vi "getAllChannels.vi"(8 "error in (no error)":errorcluster, 11 "Inst.Krohn-Hite-7008 in":refnum<class "Inst.Krohn-Hite-7008.lvclass">) -> (0 "error out":errorcluster, 2 "allChannelProperties":T1 {"channel" min=1 max=8 step=1}, 3 "Inst.Krohn-Hite-7008 out":refnum<class "Inst.Krohn-Hite-7008.lvclass">)   [LabVIEW 2019, in "Inst.Krohn-Hite-7008.lvclass"]
uses:
  Inst.Krohn-Hite-7008.lvclass
  C:/Program Files (x86)/National Instruments/LabVIEW 2019/user.lib/LevyLab/Instrument Framework/SMOs/Instrument/Instrument.lvclass
  KH7008/typedefs/allChannelProperties--Array.ctl
  KH7008/typedefs/channelProperties--Cluster.ctl
  KH7008/typedefs/channel--numeric.ctl
  KH7008/typedefs/gain--enum.ctl
  KH7008/typedefs/Input--Enum.ctl
  KH7008/typedefs/shunt--enum.ctl
  KH7008/typedefs/couple--Enum.ctl
  KH7008/typedefs/Filter--Enum.ctl
  Typedefs/Inst.Krohn-Hite-7008.PublicCommands--Enum.ctl
  Typedefs/getAllChannelsResponse--Cluster.ctl
  <userlib>/LevyLab/Instrument Framework/SMOs/Instrument/Instrument.lvclass/Instrument.ctl
  38ca2375-f501-4891-9a0c-4469223ebde2.vi
  38ca2375-f501-4891-9a0c-4469223ebde2.vi/5aa567ac-1695-459b-a1d0-b3af6574eea6.vi
  <userlib>/LevyLab/Instrument Framework/SMOs/Instrument/API/Send and Receive.vi
  38ca2375-f501-4891-9a0c-4469223ebde2.vi/e3c320c6-cd25-45d0-953c-8e0f206248d2.vi
  <userlib>/LevyLab/Instrument Framework/SMOs/Instrument/Private/Get Client Type.vi
  38ca2375-f501-4891-9a0c-4469223ebde2.vi/5aa567ac-1695-459b-a1d0-b3af6574eea6.vi/1d0ba0ad-da3a-4e7e-a3ed-5df425220c22.vi
  38ca2375-f501-4891-9a0c-4469223ebde2.vi/5aa567ac-1695-459b-a1d0-b3af6574eea6.vi/db69f284-e81f-4a99-80b8-8d5d4eb5535a.vi
  38ca2375-f501-4891-9a0c-4469223ebde2.vi/e3c320c6-cd25-45d0-953c-8e0f206248d2.vi/5e0845a0-105c-47ce-984f-8bb23b57a8af.vi
  38ca2375-f501-4891-9a0c-4469223ebde2.vi/e3c320c6-cd25-45d0-953c-8e0f206248d2.vi/63a6940b-2958-4188-9028-e5d62b597068.vi
  38ca2375-f501-4891-9a0c-4469223ebde2.vi/e3c320c6-cd25-45d0-953c-8e0f206248d2.vi/5e0845a0-105c-47ce-984f-8bb23b57a8af.vi/888d27de-f54c-4ced-8122-603733a70d87.vi
  38ca2375-f501-4891-9a0c-4469223ebde2.vi/e3c320c6-cd25-45d0-953c-8e0f206248d2.vi/5e0845a0-105c-47ce-984f-8bb23b57a8af.vi/d37ea9d1-0233-473e-ac15-01733ff54870.vi
  <userlib>/LevyLab/Instrument Framework/SMOs/Instrument/Private/Get RC Connection Status.vi
  <userlib>/LevyLab/Instrument Framework/SMOs/Instrument/API/Enum to String.vi
  <userlib>/LevyLab/Instrument Framework/SMOs/RemoteControl/API/Send and Receive.vi
  <vilib>/Utility/Data Type/Get Type Information.vi
  <vilib>/JDP Science/JSONtext/JSON text to Variant.vi
  <userlib>/LevyLab/Instrument Framework/SMOs/Instrument/API/Instrument.GetPublicEvents.vi
  <vilib>/JDP Science/JSONtext/Variant to JSON Text.vi
  <vilib>/National Instruments/GUID Generator/Guid Generator.vi
  <userlib>/LevyLab/Instrument Framework/SMOs/Instrument/API/Instrument.MessageToProcess.vi
  <userlib>/LevyLab/Instrument Framework/SMOs/Instrument/Private/Instrument.MessageFromProcess.EventStructure.vi
  <vilib>/JDP Science/JSONtext/LVClass Serializer/JSONtext LVClass Serializer.lvclass
  KH7008/KH7008.lvlib
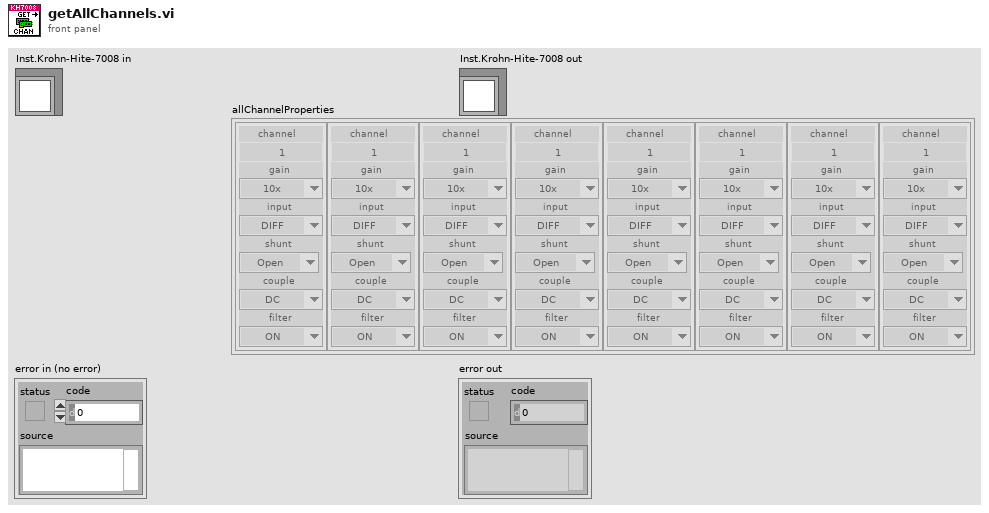
[diagram p1: front panel]
types:
  T1 = typedef "KH7008.lvlib/allChannelProperties--Array.ctl" = T2[]
  T2 = typedef "KH7008.lvlib/channelProperties--Cluster.ctl" = cluster{"channel":T3, "gain":T4, "input":T5, "shunt":T6, "couple":T7, "filter":T8}
  T3 = typedef "KH7008.lvlib/channel--numeric.ctl" = u16
  T4 = typedef "KH7008.lvlib/gain--enum.ctl" = enum16{"1x", "10x", "100x", "1000x"}
  T5 = typedef "KH7008.lvlib/input--enum.ctl" = enum16{"OFF", "SE+", "SE-", "DIFF"}
  T6 = typedef "KH7008.lvlib/shunt--enum.ctl" = enum16{"Open", "50", "500", "5k", "50k", "10M"}
  T7 = typedef "KH7008.lvlib/couple--enum.ctl" = enum16{"AC", "DC"}
  T8 = typedef "KH7008.lvlib/filter--enum.ctl" = enum16{"OFF", "ON"}
  T9 = typedef "Inst.Krohn-Hite-7008.lvclass/getAllChannelsResponse--Cluster.ctl" = cluster{"allChannelProperties":T1}
  T10 = typedef "Inst.Krohn-Hite-7008.lvclass/Inst.Krohn-Hite-7008.PublicCommands--Enum.ctl" = enum16{"getChannel", "getAllChannels", "setChannel", "setAllChannels"}
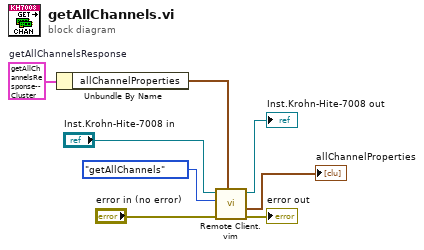
[diagram p0: block diagram]
diagram:
  w3 = T9 {"allChannelProperties"=[{"channel"=1, "gain"=enum."10x", "input"=enum."OFF", "shunt"=enum."10M", "couple"=enum."AC", "filter"=enum."OFF"}, {"channel"=2, "gain"=enum."10x", "input"=enum."OFF", "shunt"=enum."10M", "couple"=enum."AC", "filter"=enum."OFF"}, {"channel"=3, "gain"=enum."10x", "input"=enum."OFF", "shunt"=enum."10M", "couple"=enum."AC", "filter"=enum."OFF"}, {"channel"=4, "gain"=enum."10x", "input"=enum."OFF", "shunt"=enum."10M", "couple"=enum."AC", "filter"=enum."OFF"}, {"channel"=5, "gain"=enum."10x", "input"=enum."OFF", "shunt"=enum."10M", "couple"=enum."AC", "filter"=enum."OFF"}, {"channel"=6, "gain"=enum."10x", "input"=enum."OFF", "shunt"=enum."10M", "couple"=enum."AC", "filter"=enum."OFF"}, {"channel"=7, "gain"=enum."10x", "input"=enum."OFF", "shunt"=enum."10M", "couple"=enum."AC", "filter"=enum."OFF"}, {"channel"=7, "gain"=enum."10x", "input"=enum."OFF", "shunt"=enum."10M", "couple"=enum."AC", "filter"=enum."OFF"}]}  # getAllChannelsResponse
  n1 = Unbundle By Name(w3) -> ("allChannelProperties"=w2:T1)
  n2 = call "Remote Client.vim"("Data Out type"=w2, "error in (no error)"="error in (no error)", "method"=Inst.Krohn-Hite-7008.PublicCommands--Enum."getAllChannels" ("publicCommands"), "Instrument in"="Inst.Krohn-Hite-7008 in") -> ("error out"=→"error out":errorcluster, "Data out"=→"allChannelProperties":T2[], "Instrument out"=→"Inst.Krohn-Hite-7008 out":refnum<class "Inst.Krohn-Hite-7008.lvclass">)  [unwired: 4 in, 1 out]
